vi "CRYSet Export TextFormat Front Panel.vi"(11 "Vi Ref":refnum<vi>) -> ()   [LabVIEW 2013]
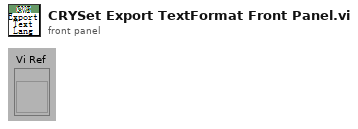
[diagram p1: front panel]
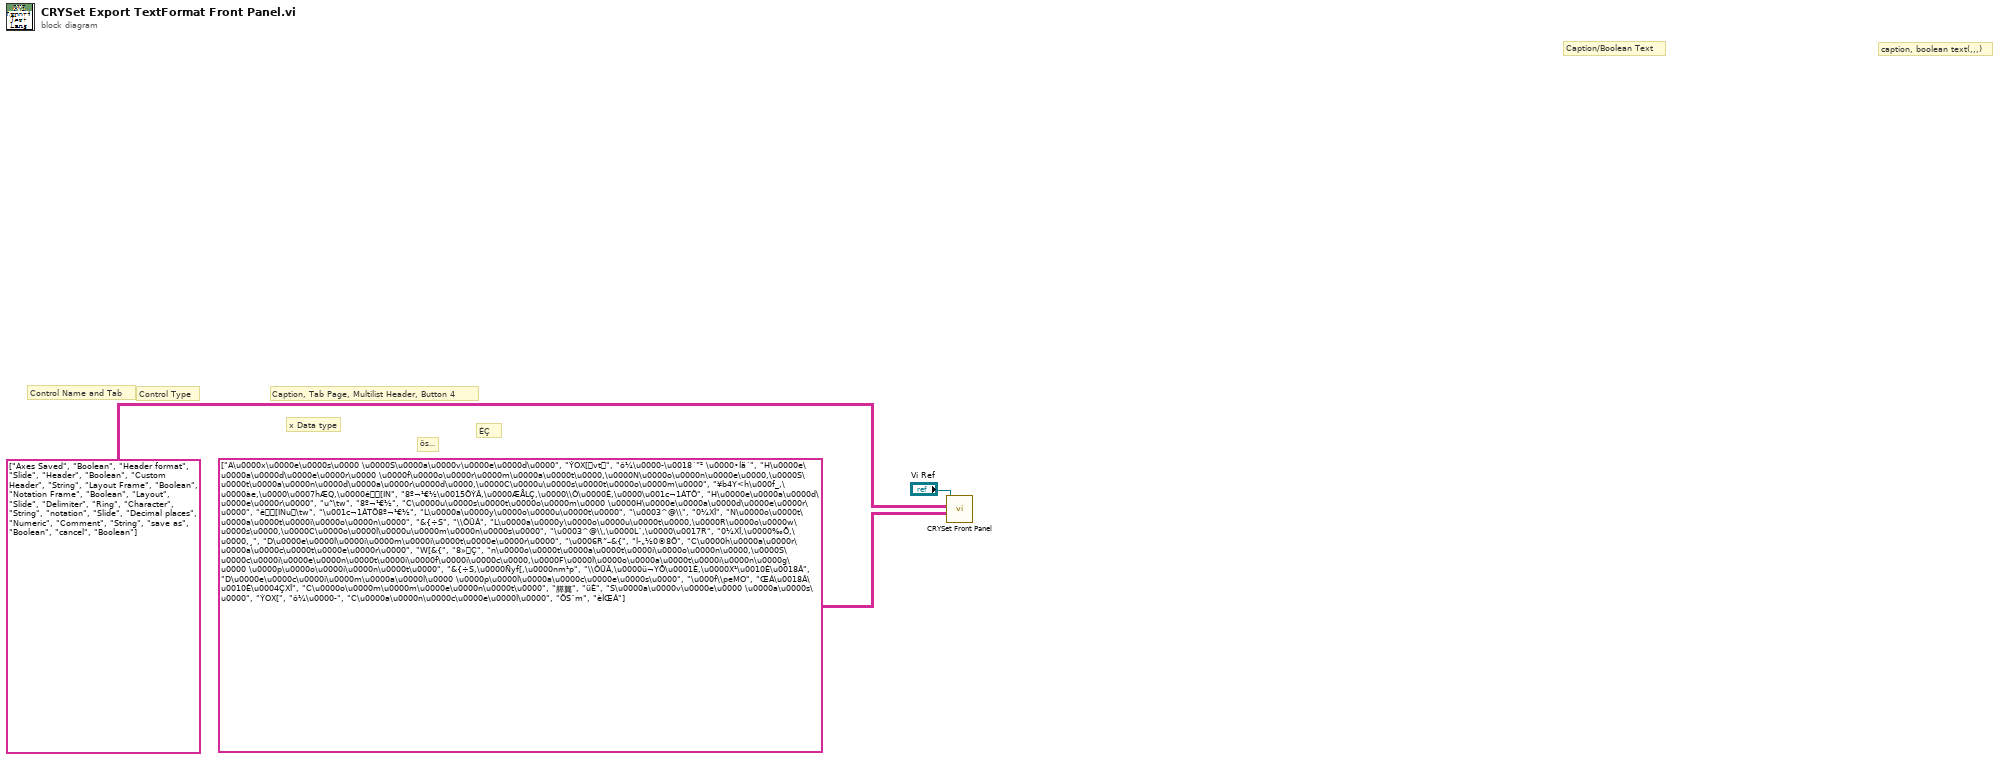
[diagram p0: block diagram]
diagram:
  # "ÉÇ"
  # "ÖSˆm"
  # "x Data type"
  # "Caption, Tab Page, Multilist Header, Button 4"
  # "Control Type"
  # "Control Name and Tab"
  # "caption, boolean text(,,,)"
  # "Caption/Boolean Text"
  n1 = call "CRYSet Front Panel.vi"("Caption(Boolean Text)"=string[][] [["A\u0000x\u0000e\u0000s\u0000 \u0000S\u0000a\u0000v\u0000e\u0000d\u0000", "ÝOX[vt", "ô¼\u0000­\u0018´”² \u0000•Íä´"], ["H\u0000e\u0000a\u0000d\u0000e\u0000r\u0000 \u0000f\u0000o\u0000r\u0000m\u0000a\u0000t\u0000,\u0000N\u0000o\u0000n\u0000e\u0000,\u0000S\u0000t\u0000a\u0000n\u0000d\u0000a\u0000r\u0000d\u0000,\u0000C\u0000u\u0000s\u0000t\u0000o\u0000m\u0000", "¥b4Y<h\u000f_,\u0000àe,\u0000\u0007hÆQ,\u0000ê[IN", "8º¬¹€½\u0015ÖÝÂ,\u0000ÆÅLÇ,\u0000\\Ô\u0000É,\u0000\u001c¬1ÁTÖ"], ["H\u0000e\u0000a\u0000d\u0000e\u0000r\u0000", "u˜\tw", "8º¬¹€½"], ["C\u0000u\u0000s\u0000t\u0000o\u0000m\u0000 \u0000H\u0000e\u0000a\u0000d\u0000e\u0000r\u0000", "ê[INu\tw", "\u001c¬1ÁTÖ8º¬¹€½"], ["L\u0000a\u0000y\u0000o\u0000u\u0000t\u0000", "\u0003^@\\", "0¼XÎ"], ["N\u0000o\u0000t\u0000a\u0000t\u0000i\u0000o\u0000n\u0000", "&{÷S", "\\ÔÜÂ"], ["L\u0000a\u0000y\u0000o\u0000u\u0000t\u0000,\u0000R\u0000o\u0000w\u0000s\u0000,\u0000C\u0000o\u0000l\u0000u\u0000m\u0000n\u0000s\u0000", "\u0003^@\\,\u0000Lˆ,\u0000\u0017R", "0¼XÎ,\u0000‰Õ,\u0000,¸"], ["D\u0000e\u0000l\u0000i\u0000m\u0000i\u0000t\u0000e\u0000r\u0000", "\u0006R”–&{", "l­„½0®8Ö"], ["C\u0000h\u0000a\u0000r\u0000a\u0000c\u0000t\u0000e\u0000r\u0000", "W[&{", "8»Ç"], ["n\u0000o\u0000t\u0000a\u0000t\u0000i\u0000o\u0000n\u0000,\u0000S\u0000c\u0000i\u0000e\u0000n\u0000t\u0000i\u0000f\u0000i\u0000c\u0000,\u0000F\u0000l\u0000o\u0000a\u0000t\u0000i\u0000n\u0000g\u0000 \u0000p\u0000o\u0000i\u0000n\u0000t\u0000", "&{÷S,\u0000Ñyf[,\u0000nm¹p", "\\ÔÜÂ,\u0000ü¬YÕ\u0001È,\u0000X¹\u0010È\u0018Â"], ["D\u0000e\u0000c\u0000i\u0000m\u0000a\u0000l\u0000 \u0000p\u0000l\u0000a\u0000c\u0000e\u0000s\u0000", "\u000f\\peMO", "ŒÁ\u0018Â\u0010È\u0004ÇXÎ"], ["C\u0000o\u0000m\u0000m\u0000e\u0000n\u0000t\u0000", "膵簨", "üÈ"], ["S\u0000a\u0000v\u0000e\u0000 \u0000a\u0000s\u0000", "ÝOX[", "ô¼\u0000­"], ["C\u0000a\u0000n\u0000c\u0000e\u0000l\u0000", "ÖSˆm", "èÍŒÁ"]], "Control ID and Type(Label Name, Type)"=string[][] [["Axes Saved", "Boolean"], ["Header format", "Slide"], ["Header", "Boolean"], ["Custom Header", "String"], ["Layout Frame", "Boolean"], ["Notation Frame", "Boolean"], ["Layout", "Slide"], ["Delimiter", "Ring"], ["Character", "String"], ["notation", "Slide"], ["Decimal places", "Numeric"], ["Comment", "String"], ["save as", "Boolean"], ["cancel", "Boolean"]], "Vi Ref"="Vi Ref") -> ()  [unwired: 9 in]
